vi "Base64url_Add_Padding.vi"(1 "Base64url string":string) -> (0 "Base64 string":string)   [LabVIEW 2013, in "Serializer.Base64.lvclass"]
doc: "Adds padding (up to two \"=\" chars) to Base64url string to allow for decoding.\n\nPer RFC, Base64url strings <B>MAY</B> be unpadded. The CORE decoding VI\nrequires padding to properly decode."
uses:
  Serializer.Base64.lvclass
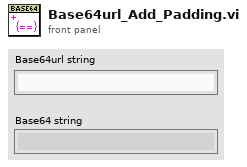
[diagram p1: front panel]
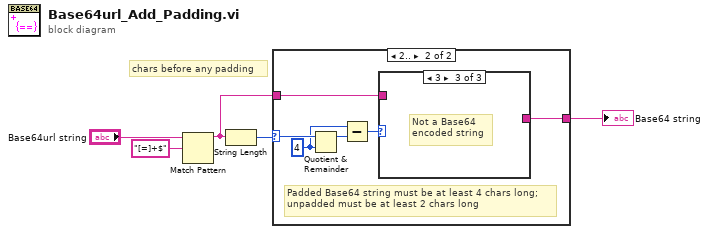
[diagram p0: block diagram]
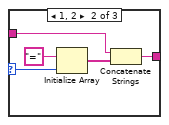
[diagram p4: hidden frame]
diagram:
  # "chars before any padding"
  n1 = Match Pattern(string="Base64url string", regular expression="[=]+$") -> (before substring=w2:string)  [unwired: 1 in, 3 out]
  n2 = String Length(string=w2) -> (length=w3:i32)
  n3 = case shown="2.." w3 {
    selector: w3 -> [_ w11]
    tunnel: w2 -> [_ w7]
    tunnel: [_ w6] -> w1
    frame ..1, Default {
    }
    frame 2.. {
      w9 = 4 ("y")
      # "Padded Base64 string must be at least 4 chars long;\nunpadded must be at least 2 chars long"
      n4 = Quotient & Remainder(x=w11, y=w9) -> (x-y*floor(x/y)=w8:i32)  [unwired: 1 out]
      n5 = Subtract(x=w9, y=w8) -> (x-y=w10:i32)
      n6 = case shown="3" w10 {
        selector: w10 -> [_ w16 _]
        tunnel: w7 -> [w12 w15 _]
        tunnel: [w12 w13 _] -> w6
        frame 0, Default {
        }
        frame 1, 2 {
          n7 = Initialize Array("=", w16) -> (w14:string[])
          n8 = Concatenate Strings(w15, w14) -> (w13:string)
        }
        frame 3 {
          # "Not a Base64\nencoded string"
        }
      }
    }
  }
  "Base64 string" <- w1
